vi "Constructor.vi"(8 "error in":errorcluster, 10 "WindowTitle":string, 11 "WindowFrame in":refnum<class "WindowFrame.lvclass">) -> (0 "error out":errorcluster, 2 "WindowFrame":refnum<event-registration>, 3 "WindowFrame out":refnum<class "WindowFrame.lvclass">)   [LabVIEW 2021, in "WindowFrame.lvlib" / "WindowFrame.lvclass"]
uses:
  WindowFrame.lvclass
  WindowFrame.lvclass/WindowFrame.ctl
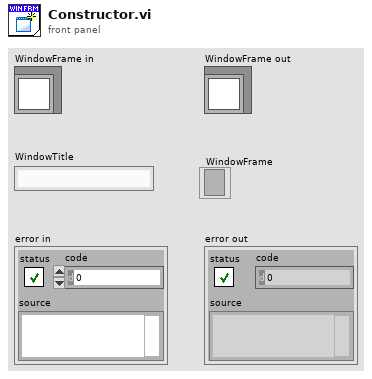
[diagram p1: front panel]
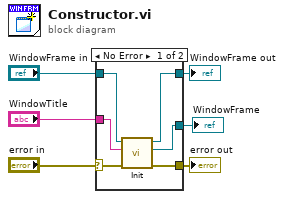
[diagram p0: block diagram]
diagram:
  n1 = case shown="No Error" "error in" {
    selector: "error in" -> [w11 w14]
    tunnel: [w10 w14] -> w6
    tunnel: [w8 w13] -> w3
    tunnel: "WindowFrame in" -> [w12 w13]
    tunnel: "WindowTitle" -> [w9 _]
    tunnel: [w7 _] -> w1
    frame No Error {
      n2 = call "Init.vi"("error in (no error)"=w11, "WindowTitle"=w9, "WindowFrame in"=w12) -> ("error out"=w10:errorcluster, "WindowFrame"=w7:refnum<event-registration>, "WindowFrame out"=w8:refnum<class "WindowFrame.lvclass">)  [unwired: 6 in]
    }
    frame Error {
    }
  }
  "WindowFrame out" <- w3
  "error out" <- w6
  "WindowFrame" <- w1
